vi "Create a New Run.vi"(7 "xwpfRun Type":refnum<class "xwpfRun.lvclass">, 8 "error in (no error)":errorcluster, 9 "Style":refnum<class "Style.lvclass">, 10 "Text":string, 11 "Run Ref":refnum<k24>) -> (0 "error out":errorcluster, 3 "xwpfRun out":refnum<class "xwpfRun.lvclass">)   [LabVIEW 2017, in "Word_Specific.lvlib" / "xwpfRun.lvclass"]
uses:
  xwpfRun.lvclass
  Styles/Style/Style.lvclass
  C:/Users/Neo/Desktop/Dev_Tools_BR/LabVIEW_NPOI/src/lib/NPOI 2.1.1/NPOI.OOXML.dll
  lib/NPOI 2.1.1/NPOI.OOXML.dll
  xwpfRun.lvclass/xwpfRun.ctl
  Set Style.vi
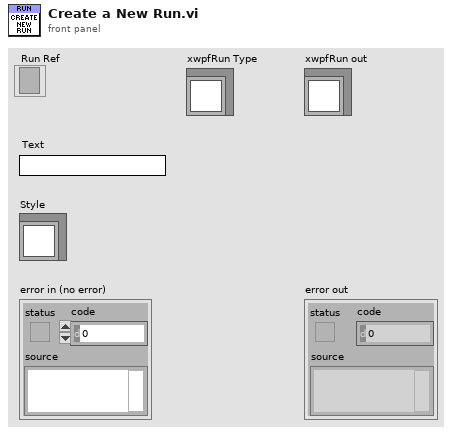
[diagram p1: front panel]
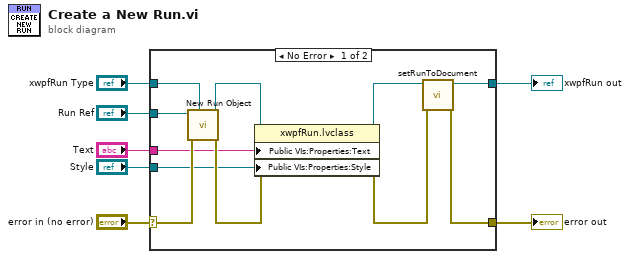
[diagram p0: block diagram]
diagram:
  n1 = case shown="No Error" "error in (no error)" {
    selector: "error in (no error)" -> [w12 w20]
    tunnel: [w11 w20] -> w6
    tunnel: [w14 w19] -> w4
    tunnel: "xwpfRun Type" -> [w18 w19]
    tunnel: "Run Ref" -> [w17 _]
    tunnel: "Text" -> [w9 _]
    tunnel: "Style" -> [w8 _]
    frame No Error {
      n2 = call "New Run Object.vi"("xwpfRun Type"=w18, "error in (no error)"=w12, "Run Ref"=w17) -> ("error out"=w16:errorcluster, "xwpfRun out"=w15:refnum<class "xwpfRun.lvclass">)  [unwired: 7 in]
      n3 = property class="xwpfRun.lvclass"(reference=w15, error in=w16, "Public VIs:Properties:Text"=w9, "Public VIs:Properties:Style"=w8) -> (reference out=w13:refnum<class "xwpfRun.lvclass">, error out=w10:errorcluster)
      n4 = call-dynamic "setRunToDocument.vi"("error in (no error)"=w10, "xwpfRun in"=w13) -> ("error out"=w11:errorcluster, "xwpfRun out"=w14:refnum<class "xwpfRun.lvclass">)  [unwired: 8 in]
    }
    frame Error {
    }
  }
  "error out" <- w6
  "xwpfRun out" <- w4
